vi "Cypher XY LVDT Parameters_Cypher.vi"() -> ()   [LabVIEW 2019]
panel:
  in  "Cypher YLVDT Offset":dbl=1.02
  in  "Cypher XLVDT Offset":dbl=-0.77
  in  "Cypher YLVDT Sens":dbl=4.5835e-06
  in  "Cypher XLVDT Sens":dbl=4.92888e-06
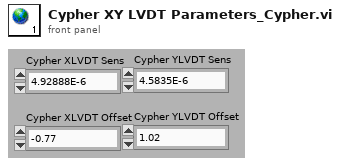
[diagram p1: front panel]
diagram:
